vi "Set line.vi"(8 "error in (no error)":errorcluster, 9 "Action":enum16{"Open", "Close", "Toggle"}(ring)=enum."Toggle", 10 "Line number":u8, 11 "TTL in":refnum<class "TTL.lvclass">) -> (0 "error out":errorcluster, 3 "TTL out":refnum<class "TTL.lvclass">)   [LabVIEW 2014, in "TTL.lvclass"]
doc: "Sets a new value on a specific line.\nIf the line is suppressed, the command is ignored."
uses:
  TTL.lvclass
  TTL.lvclass/TTL.ctl
  <vilib>/DAQmx/read.llb/DAQmx Read (Digital 1D Bool NChan 1Samp 1Line).vi
  <vilib>/DAQmx/write.llb/DAQmx Write (Digital 1D Bool NChan 1Samp 1Line).vi
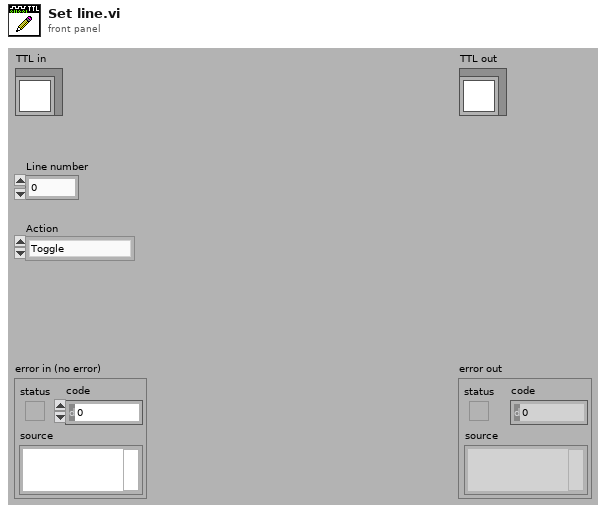
[diagram p1: front panel]
types:
  T1 = typedef "TTL.lvclass/TTL Status Data.ctl" = cluster{"Line states before suppression":bool[], "Suppressed lines":bool[]}
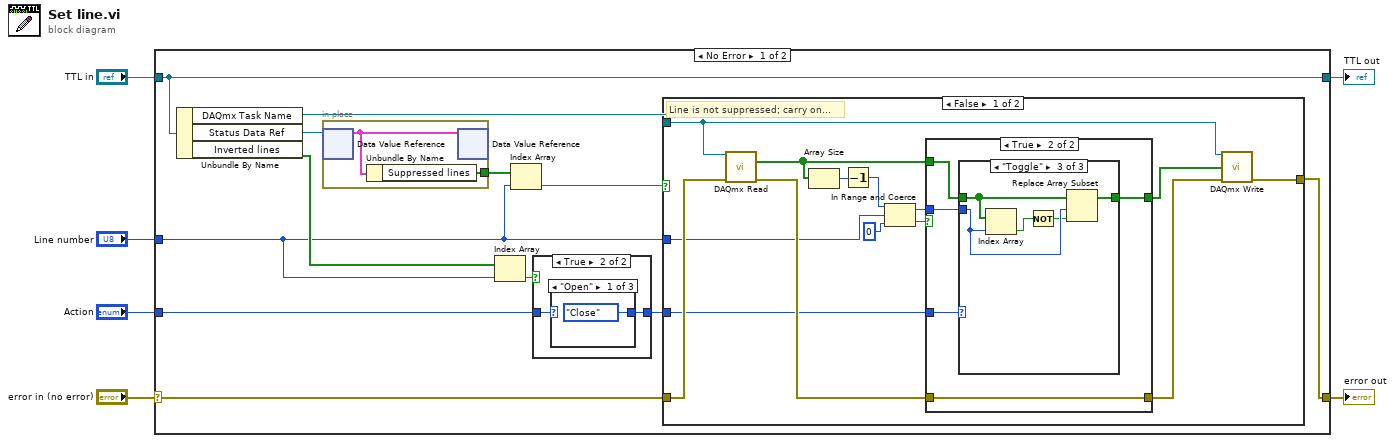
[diagram p0: block diagram]
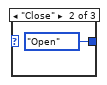
[diagram p3: hidden frame]
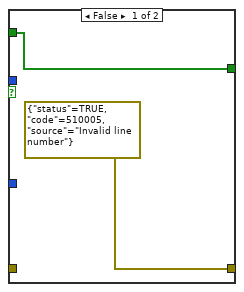
[diagram p5: hidden frame]
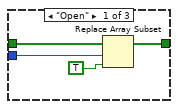
[diagram p6: hidden frame]
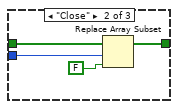
[diagram p7: hidden frame]
diagram:
  n1 = case shown="No Error" "error in (no error)" {
    selector: "error in (no error)" -> [w18 w63]
    tunnel: [w15 w63] -> w5
    tunnel: [w17 w62] -> w3
    tunnel: "TTL in" -> [w17 w62]
    tunnel: "Line number" -> [w12 _]
    tunnel: "Action" -> [w10 _]
    frame No Error {
      n2 = Unbundle By Name(w17) -> ("DAQmx Task Name"=w16:refnum<k21>, "Status Data Ref"=w8:refnum<data-value>, "Inverted lines"=w13:bool[])
      n3 = in-place {
        in-place-border: [w19] -> w7
        n4 = in-place-dvr #1(w8) -> (w20:T1)  [unwired: 1 out]
        n5 = Unbundle By Name(w20) -> ("Suppressed lines"=w19:bool[])
        n6 = in-place-dvr #1(w20) -> ()  [unwired: 2 out]
      }
      n7 = Index Array(array=w13, index=w12) -> (element=w11:bool)
      n8 = Index Array(array=w7, index=w12) -> (element=w14:bool)
      n9 = case shown="True" w11 {
        tunnel: w10 -> [w21 w23]
        tunnel: [w21 w22] -> w9
        frame False {
        }
        frame True {
          n10 = case shown="\"Open\"" w23 {
            selector: w23 -> [_ _ w26]
            tunnel: [enum16{"Open", "Close", "Toggle"}."Close" ("Action") enum16{"Open", "Close", "Toggle"}."Open" ("Action") w26] -> w22
            frame "Open" {
            }
            frame "Close" {
            }
            frame "Toggle", Default {
            }
          }
        }
      }
      n11 = case shown="False" w14 {
        tunnel: w18 -> [w40 w61]
        tunnel: w16 -> [w33 _]
        tunnel: [w30 w61] -> w15
        tunnel: w9 -> [w29 _]
        tunnel: w12 -> [w28 _]
        frame False {
          # "Line is not suppressed; carry on..."
          n12 = call-poly <vilib>:"DAQmx Read.vi"("task/channels in"=w33, "error in"=w40) -> ("data"=w34:bool[], "error out"=w39:errorcluster)  [unwired: 11 in, 1 out]
          n13 = Array Size(array=w34) -> (size(s)=w38:i32)
          n14 = Decrement(x=w38) -> (x-1=w27:i32)
          n15 = In Range and Coerce(upper limit=w27, x=w28, lower limit=0) -> (coerced(x)=w35:i32, In Range?=w36:bool)
          n16 = case shown="True" w36 {
            tunnel: w35 -> [_ w47]
            tunnel: [errorcluster {"status"=TRUE, "code"=510005, "source"="Invalid line number"} ("error out") w45] -> w31
            tunnel: [w41 w46] -> w32
            tunnel: w39 -> [_ w45]
            tunnel: w34 -> [w41 w44]
            tunnel: w29 -> [_ w43]
            frame False {
            }
            frame True {
              n17 = case shown="\"Toggle\"" w43 {
                tunnel: w47 -> [w51 w55 w60]
                tunnel: [w49 w53 w57] -> w46
                tunnel: w44 -> [w48 w52 w58]
                frame "Open" {
                  n18 = Replace Array Subset(array=w48, new element=TRUE ("new element/subarray"), index=w51) -> (w49:bool[])
                }
                frame "Close" {
                  n19 = Replace Array Subset(array=w52, new element=FALSE ("new element/subarray"), index=w55) -> (w53:bool[])
                }
                frame "Toggle" {
                  n20 = Index Array(array=w58, index=w60) -> (element=w59:bool)
                  n21 = Not(x=w59) -> (.not. x?=w56:bool)
                  n22 = Replace Array Subset(array=w58, new element=w56, index=w60) -> (w57:bool[])
                }
              }
            }
          }
          n23 = call-poly <vilib>:"DAQmx Write.vi"("task/channels in"=w33, "data"=w32, "error in"=w31) -> ("error out"=w30:errorcluster)  [unwired: 10 in, 2 out]
        }
        frame True {
          # "Line is suppressed; ignore"
        }
      }
    }
    frame Error {
    }
  }
  "error out" <- w5
  "TTL out" <- w3
